vi "pf_Get_3D-Data_3D02.vi"(7 "Aquired Image":T1, 8 "error in (no error)":errorcluster, 9 "FrameCombine_NrOfFrames":u32, 10 "FrameCombine_Enable":bool=TRUE, 11 "PealDetector_Mode":u32) -> (0 "error out":errorcluster, 1 "Quality Profile":u8[][](array[numeric]), 2 "Width Profile":u8[][](array[numeric]), 3 "Peak Profile":sgl[][](array[numeric]), 5 "Status Line":u8[][](array[numeric]))   [LabVIEW 2012, in "Photonfocus_Toolkit.lvlib"]
uses:
  <vilib>/vision/Image Controls.llb/IMAQ Image.ctl
  <vilib>/Analysis/Matrix/Numeric/Conversions/Array To Matrix - RA2.vi
  <vilib>/Analysis/Matrix/Numeric/Conversions/Matrix To Array - RM.vi
  <userlib>/Photonfocus Toolkit/Photonfocus_Toolkit.lvlib
  <vilib>/Analysis/Matrix/NI_Matrix.lvlib
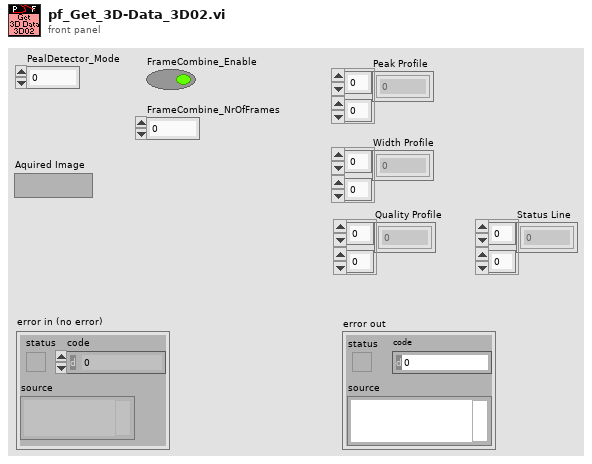
[diagram p1: front panel]
types:
  T1 = typedef "IMAQ Image.ctl" = refnum<image>
  T2 = enum8{"2D only", "2D and 3D", "3D only", "Undefined"}
  T3 = typedef "NI_Matrix.lvlib/RealMatrix.ctl" = dbl[][]
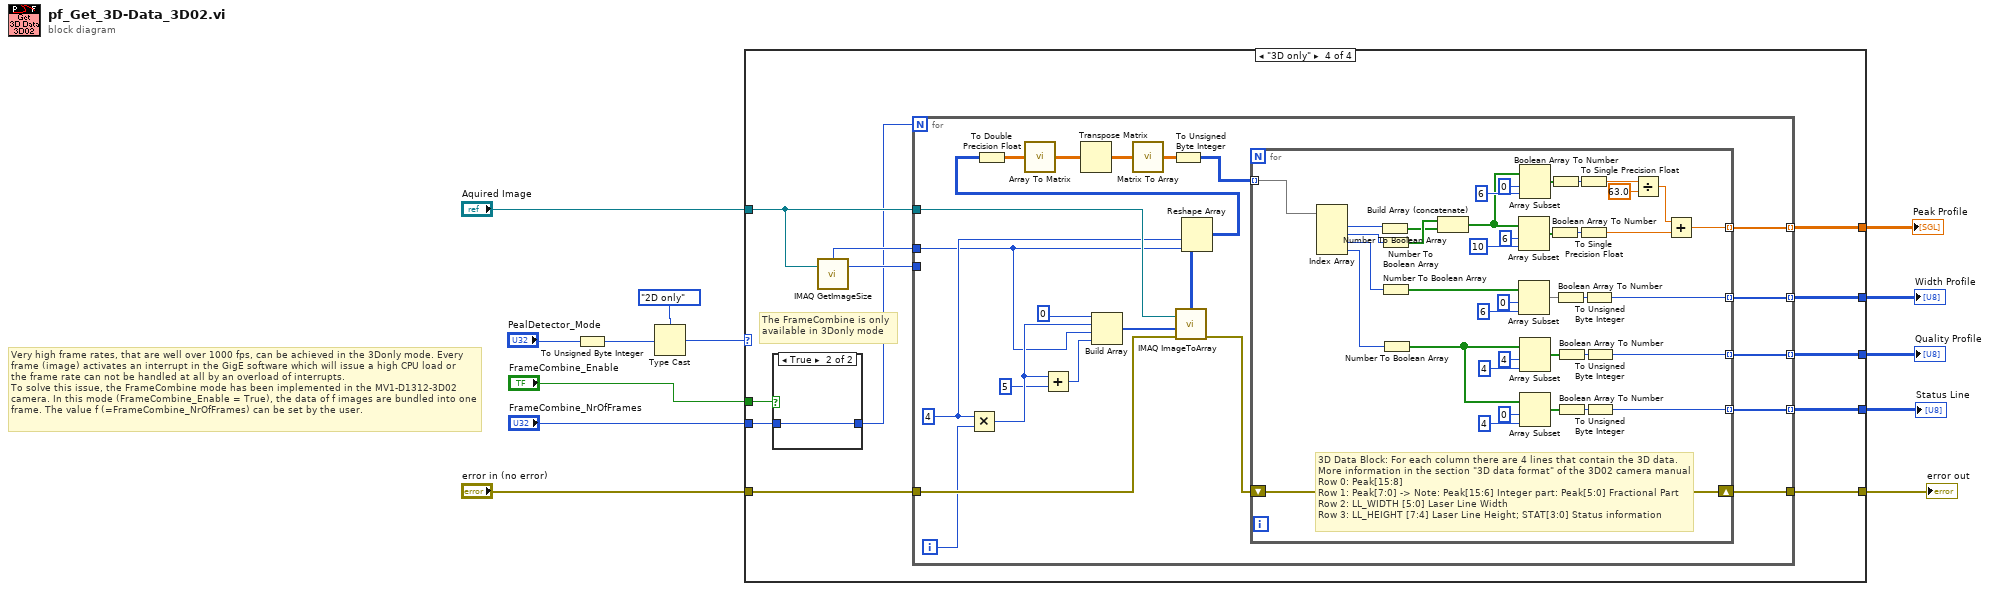
[diagram p0: block diagram]
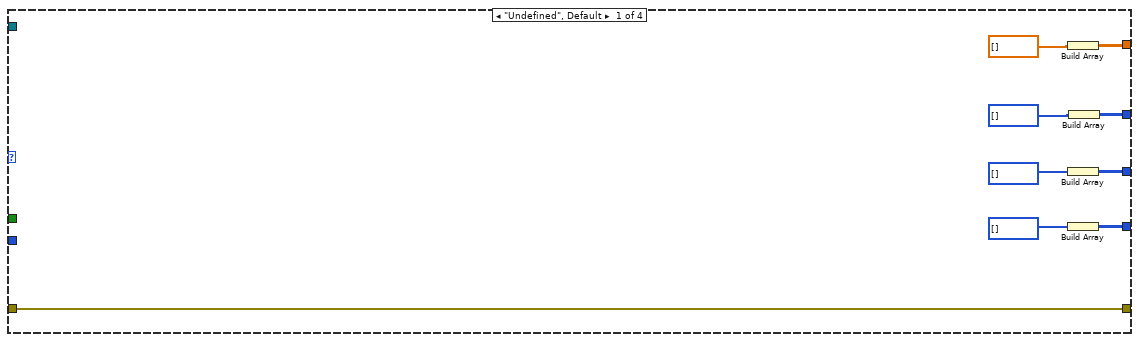
[diagram p2: hidden frame]
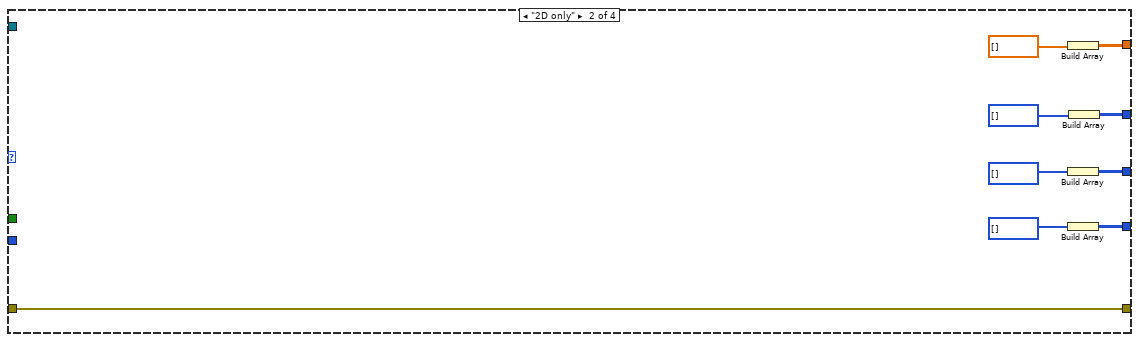
[diagram p3: hidden frame]
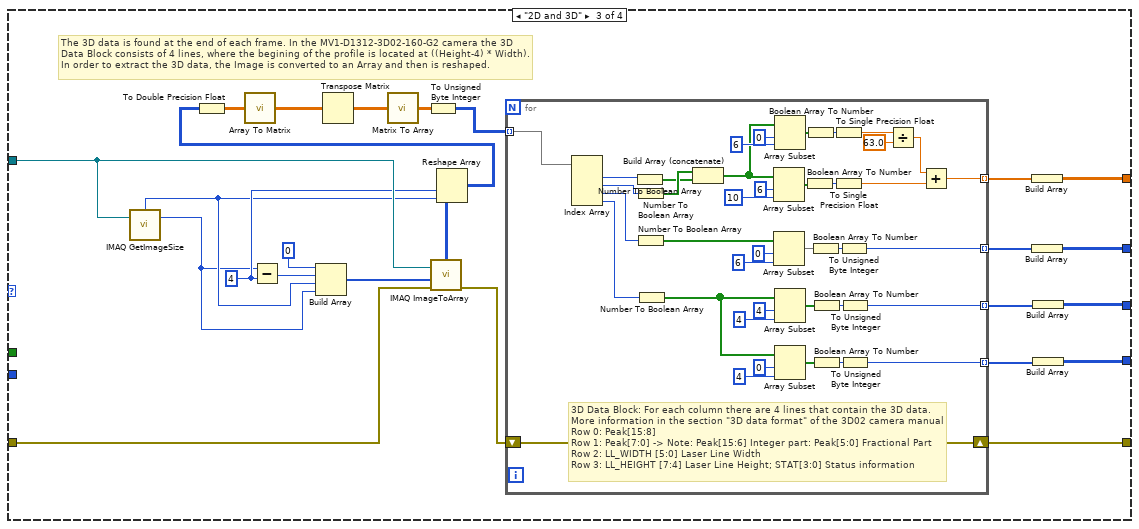
[diagram p4: hidden frame]
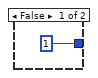
[diagram p5: hidden frame]
diagram:
  # "Very high frame rates, that are well over 1000 fps, can be achieved in the 3Donly mode. Every\nframe (image) activates an interrupt in the GigE software which will issue a high CPU load or\nthe frame rate can not be handled at all by an overload of interrupts.\nTo solve this issue, the FrameCombine mode has been implemented in the MV1-D1312-3D02\ncamera. In this mode (FrameCombine_Enable = True), the data of f images are bundled into one frame. The value f (=FrameCombine_NrOfFrames) can be set by the user."
  n1 = To Unsigned Byte Integer(number="PealDetector_Mode") -> (unsigned 8bit integer=w6:u8)
  n2 = Type Cast(type=T2."2D only", x=w6) -> (*(type *) &x=w8:T2)
  n3 = case shown="\"3D only\"" w8 {
    tunnel: "Aquired Image" -> [_ _ w49 w107]
    tunnel: [w18 w29 w40 w103] -> w4
    tunnel: [w17 w27 w38 w102] -> w3
    tunnel: [w16 w26 w36 w101] -> w2
    tunnel: [w22 w31 w55 w100] -> w12
    tunnel: "FrameCombine_NrOfFrames" -> [_ _ _ w98]
    tunnel: "error in (no error)" -> [w22 w31 w50 w104]
    tunnel: "FrameCombine_Enable" -> [_ _ _ w99]
    tunnel: [w14 w23 w34 w96] -> w1
    frame "Undefined", Default {
      n4 = Build Array(sgl[] []) -> (w18:sgl[][])
      n5 = Build Array(u8[] []) -> (w16:u8[][])
      n6 = Build Array(u8[] []) -> (w14:u8[][])
      n7 = Build Array(u8[] []) -> (w17:u8[][])
    }
    frame "2D only" {
      n8 = Build Array(sgl[] []) -> (w29:sgl[][])
      n9 = Build Array(u8[] []) -> (w26:u8[][])
      n10 = Build Array(u8[] []) -> (w23:u8[][])
      n11 = Build Array(u8[] []) -> (w27:u8[][])
    }
    frame "2D and 3D" {
      w48 = 4 ("y")
      # "The 3D data is found at the end of each frame. In the MV1-D1312-3D02-160-G2 camera the 3D Data Block consists of 4 lines, where the begining of the profile is located at ((Height-4) * Width). In order to extract the 3D data, the Image is converted to an Array and then is reshaped."
      n12 = call "IMAQ GetImageSize"("Image"=w49) -> ("Y Resolution"=w32:i32, "X Resolution"=w33:i32)  [unwired: 3 in, 1 out]
      n13 = Subtract(x=w32, y=w48) -> (x-y=w53:i32)
      n14 = Build Array "Build Array"(0, w53, w33, w32) -> (w51:i32[])
      n15 = call "IMAQ ImageToArray"("error in (no error)"=w50, "Optional Rectangle"=w51, "Image"=w49) -> ("error out"=w56:errorcluster, "Image Pixels (U8)"=w52:u8[][])  [unwired: 4 out]
      n16 = Reshape Array "Reshape Array"(w52, w48, w33) -> (w45:u8[][])
      n17 = To Double Precision Float(number=w45) -> (double precision float=w44:dbl[][])
      n18 = call-poly <vilib>:"Array To Matrix.vi"("Real 2D Array"=w44) -> ("Real Matrix"=w47:T3)
      n19 = Transpose Matrix(1:w47) -> (0:w46:T3)
      n20 = call-poly <vilib>:"Matrix To Array.vi"("Real Matrix"=w46) -> ("Real 2D Array"=w42:dbl[][])
      n21 = To Unsigned Byte Integer(number=w42) -> (unsigned 8bit integer=w43:u8[][])
      n22 = for {
        shift-right: [w71] -> w55
        shift-left: w56 -> [w71]
        tunnel: [w72] -> w41 mode=indexing
        tunnel: w43 -> [w70] mode=indexing
        tunnel: [w69] -> w39 mode=indexing
        tunnel: [w63] -> w37 mode=indexing
        tunnel: [w57] -> w35 mode=indexing
        # "3D Data Block: For each column there are 4 lines that contain the 3D data.\nMore information in the section \"3D data format\" of the 3D02 camera manual\nRow 0: Peak[15:8]\nRow 1: Peak[7:0] -> Note: Peak[15:6] Integer part: Peak[5:0] Fractional Part\nRow 2: LL_WIDTH [5:0] Laser Line Width\nRow 3: LL_HEIGHT [7:4] Laser Line Height; STAT[3:0] Status information"
        n23 = Index Array "Index Array"(array=w70) -> (element #1=w95:u8, element #2=w94:u8, element #3=w73:u8, element #4=w65:u8)  [unwired: 4 in]
        n24 = Number To Boolean Array(number=w95) -> (Boolean array=w81:bool[])
        n25 = Number To Boolean Array(number=w94) -> (Boolean array=w82:bool[])
        n26 = Number To Boolean Array(number=w73) -> (Boolean array=w74:bool[])
        n27 = Number To Boolean Array(number=w65) -> (Boolean array=w58:bool[])
        n28 = Build Array (concatenate) "Build Array"(w82, w81) -> (w83:bool[])
        n29 = Array Subset(array=w83, index=6, length=10) -> (w88:bool[])
        n30 = Array Subset(array=w74, index=0, length=6) -> (w75:bool[])
        n31 = Array Subset "Array Subset"(array=w83, index=0, length=6) -> (w89:bool[])
        n32 = Array Subset(array=w58, index=4, length=4) -> (w66:bool[])
        n33 = Array Subset(array=w58, index=0, length=4) -> (w60:bool[])
        n34 = Boolean Array To Number(Boolean array=w88) -> (number=w84:u32)
        n35 = Boolean Array To Number(Boolean array=w89) -> (number=w86:u32)
        n36 = Boolean Array To Number(Boolean array=w75) -> (number=w76:u32)
        n37 = Boolean Array To Number(Boolean array=w66) -> (number=w64:u32)
        n38 = Boolean Array To Number(Boolean array=w60) -> (number=w59:u32)
        n39 = To Single Precision Float(number=w86) -> (single precision float=w80:sgl)
        n40 = To Single Precision Float(number=w84) -> (single precision float=w79:sgl)
        n41 = To Unsigned Byte Integer(number=w76) -> (unsigned 8bit integer=w69:u8)
        n42 = To Unsigned Byte Integer(number=w64) -> (unsigned 8bit integer=w63:u8)
        n43 = To Unsigned Byte Integer(number=w59) -> (unsigned 8bit integer=w57:u8)
        n44 = Divide(x=w80, y=sgl 63.0) -> (x/y=w85:sgl)
        n45 = Add(x=w85, y=w79) -> (x+y=w72:sgl)
      }
      n46 = Build Array(w41) -> (w40:sgl[][])
      n47 = Build Array(w39) -> (w38:u8[][])
      n48 = Build Array(w37) -> (w36:u8[][])
      n49 = Build Array(w35) -> (w34:u8[][])
    }
    frame "3D only" {
      # "The FrameCombine is only available in 3Donly mode"
      n50 = case shown="True" w99 {
        tunnel: w98 -> [_ w109]
        tunnel: [1 w109] -> w97
        frame False {
        }
        frame True {
        }
      }
      n51 = call "IMAQ GetImageSize"("Image"=w107) -> ("Y Resolution"=w105:i32, "X Resolution"=w106:i32)  [unwired: 3 in, 1 out]
      n52 = for {
        N: w97 -> [_]
        tunnel: w107 -> [w122]
        tunnel: w106 -> [w111]
        tunnel: w105 -> [_]
        tunnel: w104 -> [w121]
        tunnel: [w117] -> w100
        tunnel: [w120] -> w103 mode=indexing
        tunnel: [w119] -> w102 mode=indexing
        tunnel: [w118] -> w101 mode=indexing
        tunnel: [w112] -> w96 mode=indexing
        i -> [w116]
        w113 = 4 ("y")
        n53 = Multiply(x=w113, y=w116) -> (x*y=w114:i32)
        n54 = Add(x=w114, y=5) -> (x+y=w115:i32)
        n55 = Build Array "Build Array"(0, w114, w111, w115) -> (w129:i32[])
        n56 = call "IMAQ ImageToArray"("error in (no error)"=w121, "Optional Rectangle"=w129, "Image"=w122) -> ("error out"=w132:errorcluster, "Image Pixels (U8)"=w130:u8[][])  [unwired: 4 out]
        n57 = Reshape Array "Reshape Array"(w130, w113, w111) -> (w126:u8[][])
        n58 = To Double Precision Float(number=w126) -> (double precision float=w125:dbl[][])
        n59 = call-poly <vilib>:"Array To Matrix.vi"("Real 2D Array"=w125) -> ("Real Matrix"=w128:T3)
        n60 = Transpose Matrix(1:w128) -> (0:w127:T3)
        n61 = call-poly <vilib>:"Matrix To Array.vi"("Real Matrix"=w127) -> ("Real 2D Array"=w123:dbl[][])
        n62 = To Unsigned Byte Integer(number=w123) -> (unsigned 8bit integer=w124:u8[][])
        n63 = for {
          shift-right: [w147] -> w117
          shift-left: w132 -> [w147]
          tunnel: [w148] -> w120 mode=indexing
          tunnel: w124 -> [w146] mode=indexing
          tunnel: [w145] -> w119 mode=indexing
          tunnel: [w139] -> w118 mode=indexing
          tunnel: [w133] -> w112 mode=indexing
          # "3D Data Block: For each column there are 4 lines that contain the 3D data.\nMore information in the section \"3D data format\" of the 3D02 camera manual\nRow 0: Peak[15:8]\nRow 1: Peak[7:0] -> Note: Peak[15:6] Integer part: Peak[5:0] Fractional Part\nRow 2: LL_WIDTH [5:0] Laser Line Width\nRow 3: LL_HEIGHT [7:4] Laser Line Height; STAT[3:0] Status information"
          n64 = Index Array "Index Array"(array=w146) -> (element #1=w171:u8, element #2=w170:u8, element #3=w149:u8, element #4=w141:u8)  [unwired: 4 in]
          n65 = Number To Boolean Array(number=w171) -> (Boolean array=w157:bool[])
          n66 = Number To Boolean Array(number=w170) -> (Boolean array=w158:bool[])
          n67 = Number To Boolean Array(number=w149) -> (Boolean array=w150:bool[])
          n68 = Number To Boolean Array(number=w141) -> (Boolean array=w134:bool[])
          n69 = Build Array (concatenate) "Build Array"(w158, w157) -> (w159:bool[])
          n70 = Array Subset(array=w159, index=6, length=10) -> (w164:bool[])
          n71 = Array Subset(array=w150, index=0, length=6) -> (w151:bool[])
          n72 = Array Subset "Array Subset"(array=w159, index=0, length=6) -> (w165:bool[])
          n73 = Array Subset(array=w134, index=4, length=4) -> (w142:bool[])
          n74 = Array Subset(array=w134, index=0, length=4) -> (w136:bool[])
          n75 = Boolean Array To Number(Boolean array=w164) -> (number=w160:u32)
          n76 = Boolean Array To Number(Boolean array=w165) -> (number=w162:u32)
          n77 = Boolean Array To Number(Boolean array=w151) -> (number=w152:u32)
          n78 = Boolean Array To Number(Boolean array=w142) -> (number=w140:u32)
          n79 = Boolean Array To Number(Boolean array=w136) -> (number=w135:u32)
          n80 = To Single Precision Float(number=w162) -> (single precision float=w156:sgl)
          n81 = To Single Precision Float(number=w160) -> (single precision float=w155:sgl)
          n82 = To Unsigned Byte Integer(number=w152) -> (unsigned 8bit integer=w145:u8)
          n83 = To Unsigned Byte Integer(number=w140) -> (unsigned 8bit integer=w139:u8)
          n84 = To Unsigned Byte Integer(number=w135) -> (unsigned 8bit integer=w133:u8)
          n85 = Divide(x=w156, y=sgl 63.0) -> (x/y=w161:sgl)
          n86 = Add(x=w161, y=w155) -> (x+y=w148:sgl)
        }
      }
    }
  }
  "error out" <- w12
  "Peak Profile" <- w4
  "Width Profile" <- w3
  "Quality Profile" <- w2
  "Status Line" <- w1
